vi "CLI Demo.vi"() -> ()   [LabVIEW 2020]
doc: "Demonstration of how to use the CLI.\n\nIf LUnit CLI was installed without administrator (Windows) or root (Linux/macOS) privileges the LUnit operation is not registered with the LabVIEW CLI. Set Installed without admin rights? to add -AdditionalOperationDirectory pointing at the copy installed in vi.lib/Astemes/LUnit CLI."
panel:
  out "error out":errorcluster
  out "standard output":string
  out "command line":string
  in  "Installed without admin rights?":bool
  in  "Test Case class, lvlib or lvproj":path
  in  "Report type":enum32{"txt", "xml"}(ring)
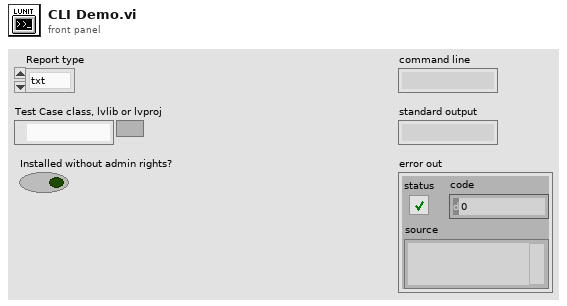
[diagram p1: front panel]
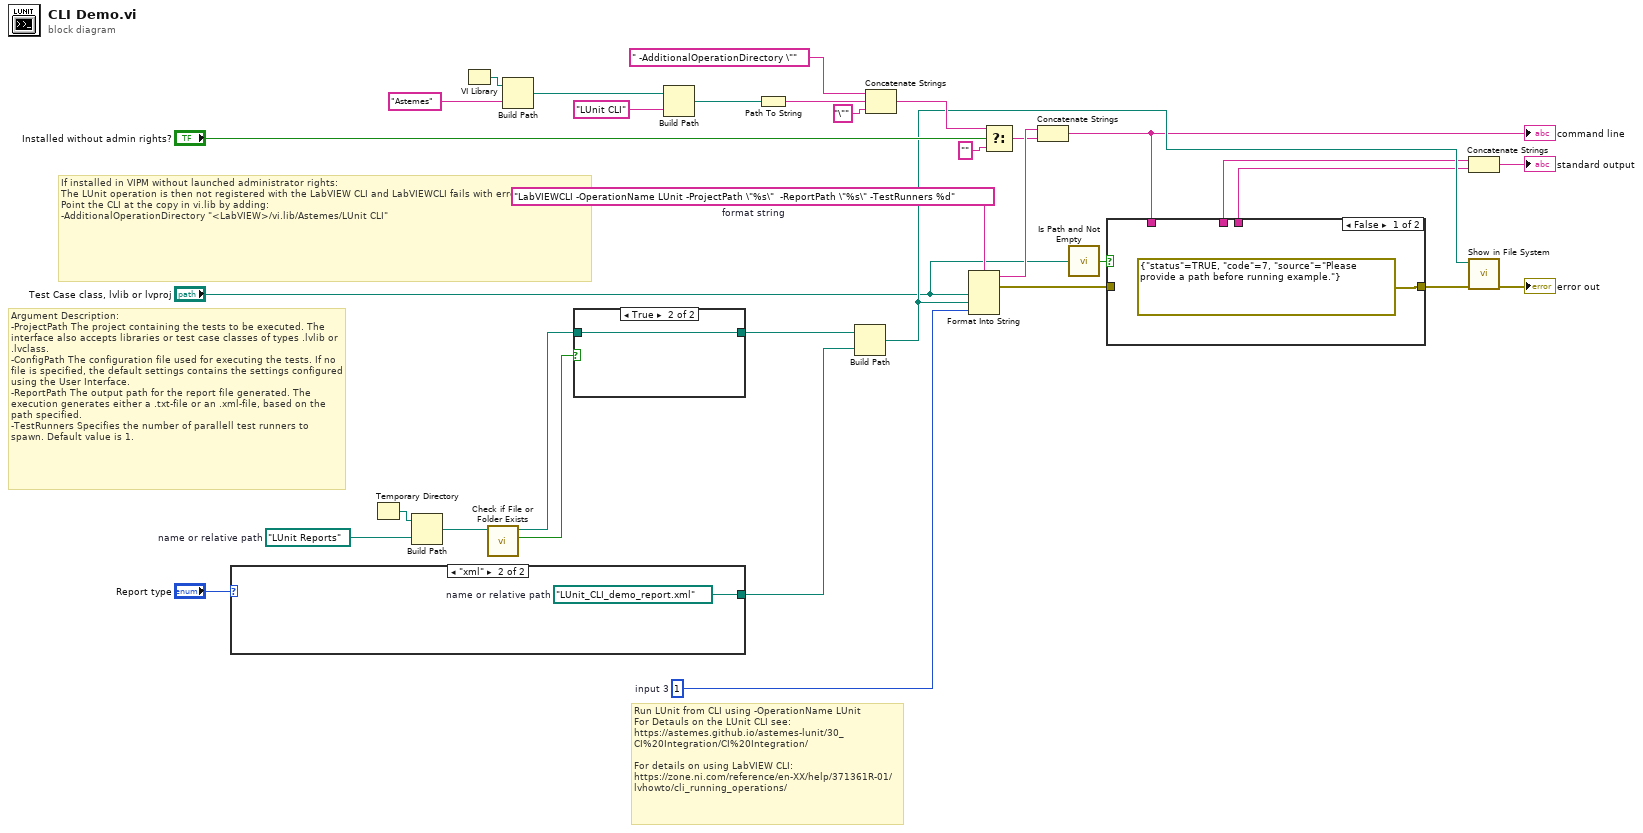
[diagram p0: block diagram]
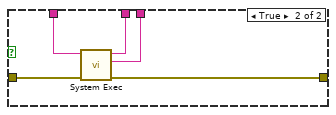
[diagram p2: hidden frame]
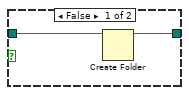
[diagram p3: hidden frame]
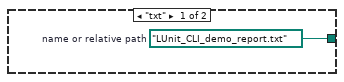
[diagram p4: hidden frame]
diagram:
  w25 = 1  # input 3
  w31 = path "LUnit Reports"  # name or relative path
  w24 = "LabVIEWCLI -OperationName LUnit -ProjectPath \"%s\"  -ReportPath \"%s\" -TestRunners %d"  # format string
  # "If installed in VIPM without launched administrator rights:\nThe LUnit operation is then not registered with the LabVIEW CLI and LabVIEWCLI fails with error -350006.\nPoint the CLI at the copy in vi.lib by adding:\n-AdditionalOperationDirectory \"<LabVIEW>/vi.lib/Astemes/LUnit CLI\""
  # "Argument\tDescription:\n-ProjectPath\tThe project containing the tests to be executed. The interface also accepts libraries or test case classes of types .lvlib or .lvclass. \n-ConfigPath\tThe configuration file used for executing the tests. If no file is specified, the default settings contains the settings configured using the User Interface.\n-ReportPath\tThe output path for the report file generated. The execution generates either a .txt-file or an .xml-file, based on the path specified.\n-TestRunners\tSpecifies the number of parallell test runners to spawn. Default value is 1."
  # "Run LUnit from CLI using -OperationName LUnit\nFor Detauls on the LUnit CLI see:\nhttps://astemes.github.io/astemes-lunit/30_CI%20Integration/CI%20Integration/\n\nFor details on using LabVIEW CLI:\nhttps://zone.ni.com/reference/en-XX/help/371361R-01/lvhowto/cli_running_operations/"
  n1 = case shown="\"xml\"" "Report type" {
    tunnel: [w34 w35] -> w26
    frame "txt" {
      w34 = path "LUnit_CLI_demo_report.txt"  # name or relative path
    }
    frame "xml" {
      w35 = path "LUnit_CLI_demo_report.xml"  # name or relative path
    }
  }
  n2 = Temporary Directory() -> (w32:path)
  n3 = Build Path(base path=w32, name or relative path=w31) -> (appended path=w30:path)
  n4 = VI Library() -> (path=w23:path)
  n5 = call <vilib>:"Check if File or Folder Exists.vi"("path"=w30) -> ("file or folder exists?"=w28:bool, "dup path"=w29:path)  [unwired: 8 in, 1 out]
  n6 = Build Path(base path=w23, name or relative path="Astemes") -> (appended path=w21:path)
  n7 = case shown="True" w28 {
    tunnel: w29 -> [w37 w38]
    tunnel: [w36 w38] -> w27
    frame False {
      n8 = Create Folder(path (use dialog)=w37) -> (created path=w36:path)  [unwired: 2 in, 2 out]
    }
    frame True {
    }
  }
  n9 = Build Path(base path=w21, name or relative path="LUnit CLI") -> (appended path=w19:path)
  n10 = Path To String(path=w19) -> (string=w17:string)
  n11 = Build Path(base path=w27, name or relative path=w26) -> (appended path=w9:path)
  n12 = Concatenate Strings(" -AdditionalOperationDirectory \"", w17, "\"") -> (w15:string)
  n13 = Format Into String(format string=w24, "Test Case class, lvlib or lvproj", w9, w25) -> (resulting string=w12:string, error out=w10:errorcluster)  [unwired: 2 in]
  n14 = Select(t=w15, s="Installed without admin rights?", f="") -> (s? t:f=w11:string)
  n15 = Concatenate Strings(w12, w11) -> (w5:string)
  "command line" <- w5
  n16 = call <vilib>:"Is Path and Not Empty.vi"("path"="Test Case class, lvlib or lvproj") -> ("Is Path and Not Empty?"=w1:bool)  [unwired: 4 in]
  n17 = case shown="False" w1 {
    tunnel: [errorcluster {"status"=TRUE, "code"=7, "source"="Please provide a path before running example."} ("error out") w44] -> w8
    tunnel: [_ w43] -> w7
    tunnel: [_ w42] -> w6
    tunnel: w5 -> [_ w41]
    tunnel: w10 -> [_ w40]
    frame False {
    }
    frame True {
      n18 = call <vilib>:"System Exec.vi"("error in (no error)"=w40, "command line"=w41) -> ("error out"=w44:errorcluster, "standard error"=w42:string, "standard output"=w43:string)  [unwired: 6 in, 1 out]
    }
  }
  n19 = Concatenate Strings(w7, w6) -> (→"standard output":string)
  n20 = call <vilib>:"Show in File System.vi"("error in (no error)"=w8, "file or directory path"=w9) -> ("error out"=→"error out":errorcluster)  [unwired: 9 in]
